vi "user32_DestroyWindow.vi"(0 "hWnd":u32, 11 "错误输入（无错误）":errorcluster) -> (4 "dup hWnd":u32, 6 "success?":bool, 15 "错误输出":errorcluster)   [LabVIEW 2011]
doc: "销毁指定的窗口。这个函数通过发送WM_DESTROY 消息和 WM_NCDESTROY 消息使窗口无效并移除其键盘焦点。这个函数还销毁窗口的菜单，清空线程的消息队列，销毁与窗口过程相关的定时器，解除窗口对剪贴板的拥有权，打断剪贴板器的查看链。"
uses:
  user32.dll
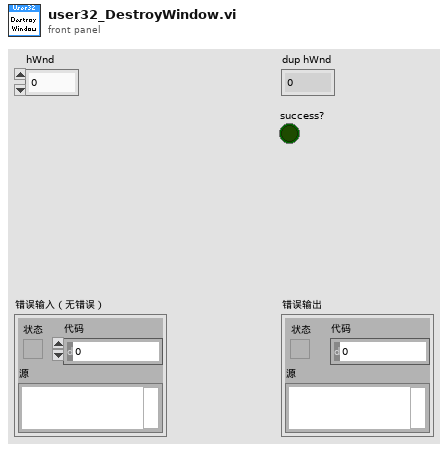
[diagram p1: front panel]
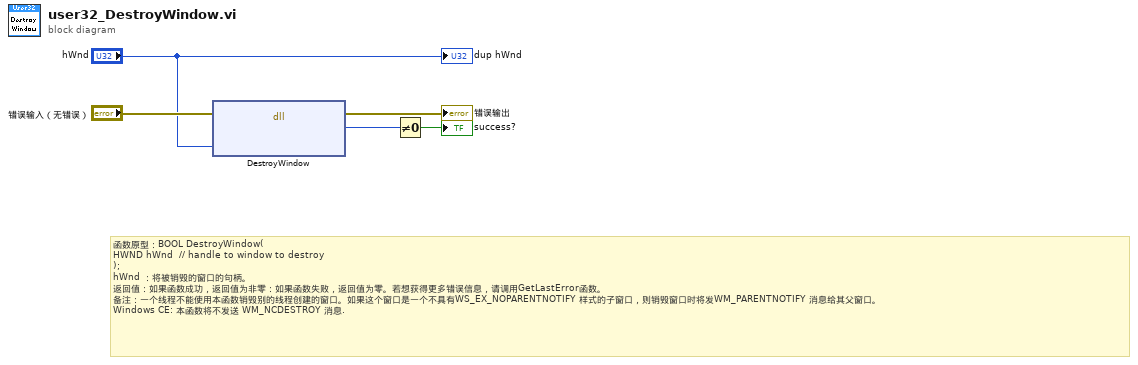
[diagram p0: block diagram]
diagram:
  # "函数原型：BOOL DestroyWindow(\nHWND hWnd  // handle to window to destroy \n);　　\nhWnd ：将被销毁的窗口的句柄。\n返回值：如果函数成功，返回值为非零：如果函数失败，返回值为零。若想获得更多错误信息，请调用GetLastError函数。\n备注：一个线程不能使用本函数销毁别的线程创建的窗口。如果这个窗口是一个不具有WS_EX_NOPARENTNOTIFY 样式的子窗口，则销毁窗口时将发WM_PARENTNOTIFY 消息给其父窗口。\nWindows CE: 本函数将不发送 WM_NCDESTROY 消息."
  n1 = dll-call lib="user32.dll" fn="DestroyWindow"(error in="错误输入（无错误）", "hWnd"="hWnd") -> (error out=→"错误输出":errorcluster, "Bool"=w2:u8)  [unwired: 3 in, 1 out]
  n2 = Not Equal To 0?(x=w2) -> (x != 0?=→"success?":bool)
  "dup hWnd" <- "hWnd"
